vi "_XNET Split Database Cluster.vi"(7 "error in (no error)":errorcluster, 10 "database cluster":string) -> (0 "error out":errorcluster, 2 "cluster":string, 3 "database":string)   [LabVIEW 2018]
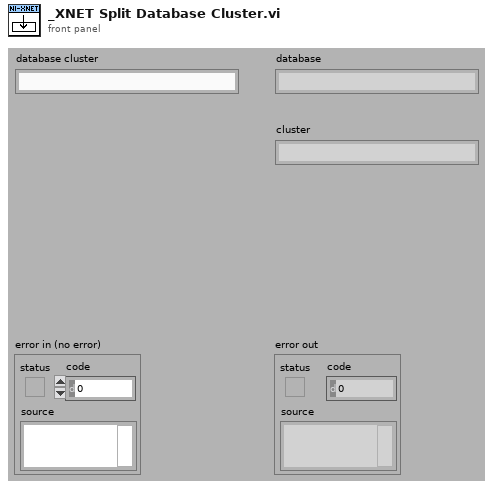
[diagram p1: front panel]
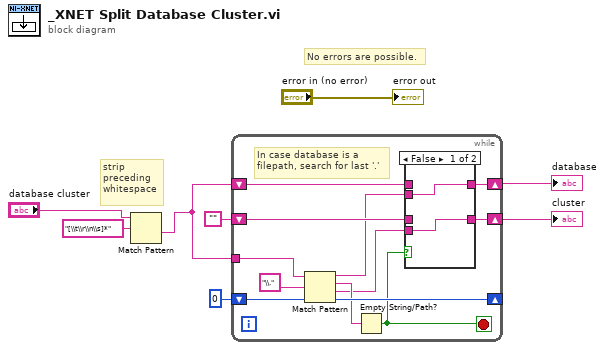
[diagram p0: block diagram]
diagram:
  # "strip\npreceding\nwhitespace"
  # "No errors are possible."
  n1 = Match Pattern(string="database cluster", regular expression="[\\t\\r\\n\\s]*") -> (after substring=w1:string)  [unwired: 4 out]
  n2 = while {
    shift-right: [w18] -> _
    shift-left: 0 ("offset (0)") -> [w19]
    shift-right: [w14] -> w7
    shift-left: w1 -> [w15]
    shift-right: [w12] -> w6
    shift-left: "" -> [w13]
    tunnel: w1 -> [w9]
    stop <- w16 stop-if-true
    # "In case database is a \nfilepath, search for last '.'"
    n3 = Match Pattern(string=w9, regular expression="\\.", offset (0)=w19) -> (before substring=w11:string, match substring=w17:string, after substring=w10:string, offset past match=w18:i32)
    n4 = Empty String/Path?(string/path=w17) -> (empty?=w16:bool)
    n5 = case shown="False" w16 {
      tunnel: w15 -> [_ w24]
      tunnel: [w22 w24] -> w14
      tunnel: w13 -> [_ w23]
      tunnel: [w21 w23] -> w12
      tunnel: w11 -> [w22 _]
      tunnel: w10 -> [w21 _]
      frame False {
      }
      frame True {
      }
    }
  }
  "database" <- w7
  "cluster" <- w6
  "error out" <- "error in (no error)"
